vi "CalStruct_View V2.vi"(8 "error in":errorcluster) -> (0 "error out":errorcluster, 2 "calbuffer":u8[](array[numeric]), 3 "Return Code":i32)   [LabVIEW 2015]
doc: "Description:\nThis function will pass a copy of the calibration structure back to a host program. The host program must be able to parse the EEPROM structure (See Appendix 1).\nDetail:\nint CalStruct_View (\nchar * calbuffer );\n\nParameters:\nchar * calbuffer - Pointer to a character buffer of bytes (needs to be able to fit the EEPROM struct data, which is currently 332 bytes), which is loaded with the local EEPROM data from the DLL.\n\nReturn Values:\nThis function returns a 0 if the function completed successfully. A non-zero return code will indicate error."
uses:
  ScannerDiagDLL.dll
panel:
  out "CalData 2":T1
  out "CalData":T1
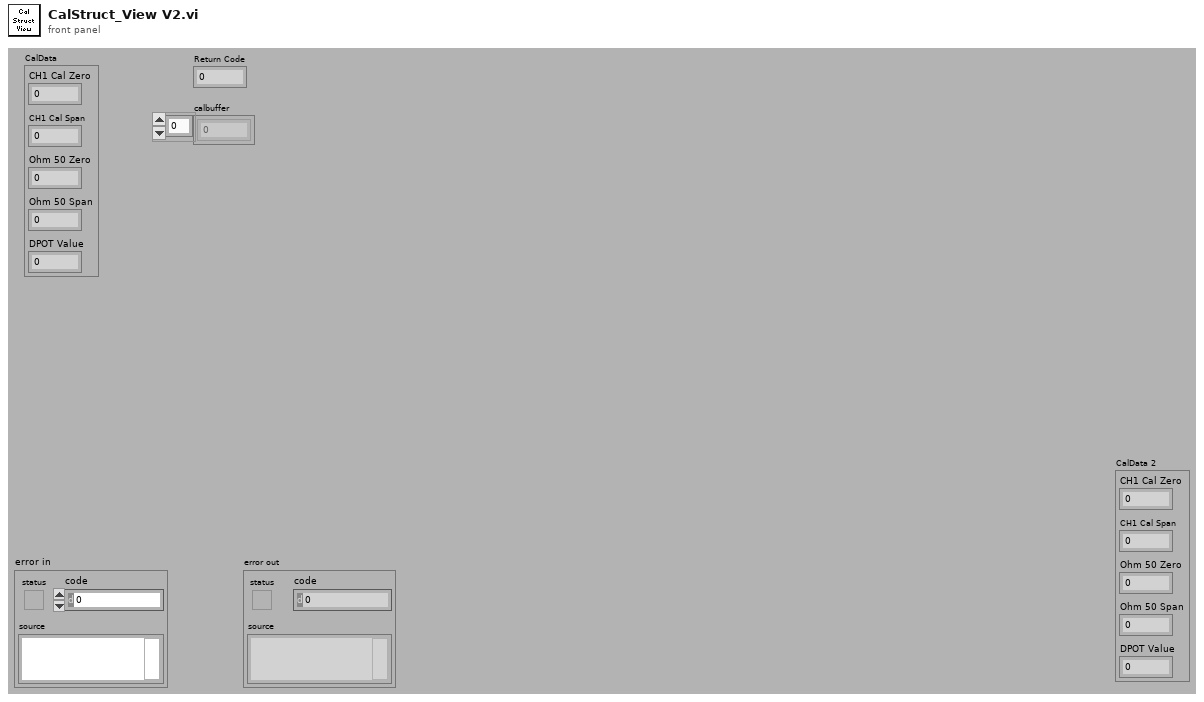
[diagram p1: front panel]
types:
  T1 = cluster{"CH1 Cal Zero ":u32, "CH1 Cal Span":u32, "Ohm 50 Zero ":u32, "Ohm 50 Span ":u32, "DPOT Value ":u32}
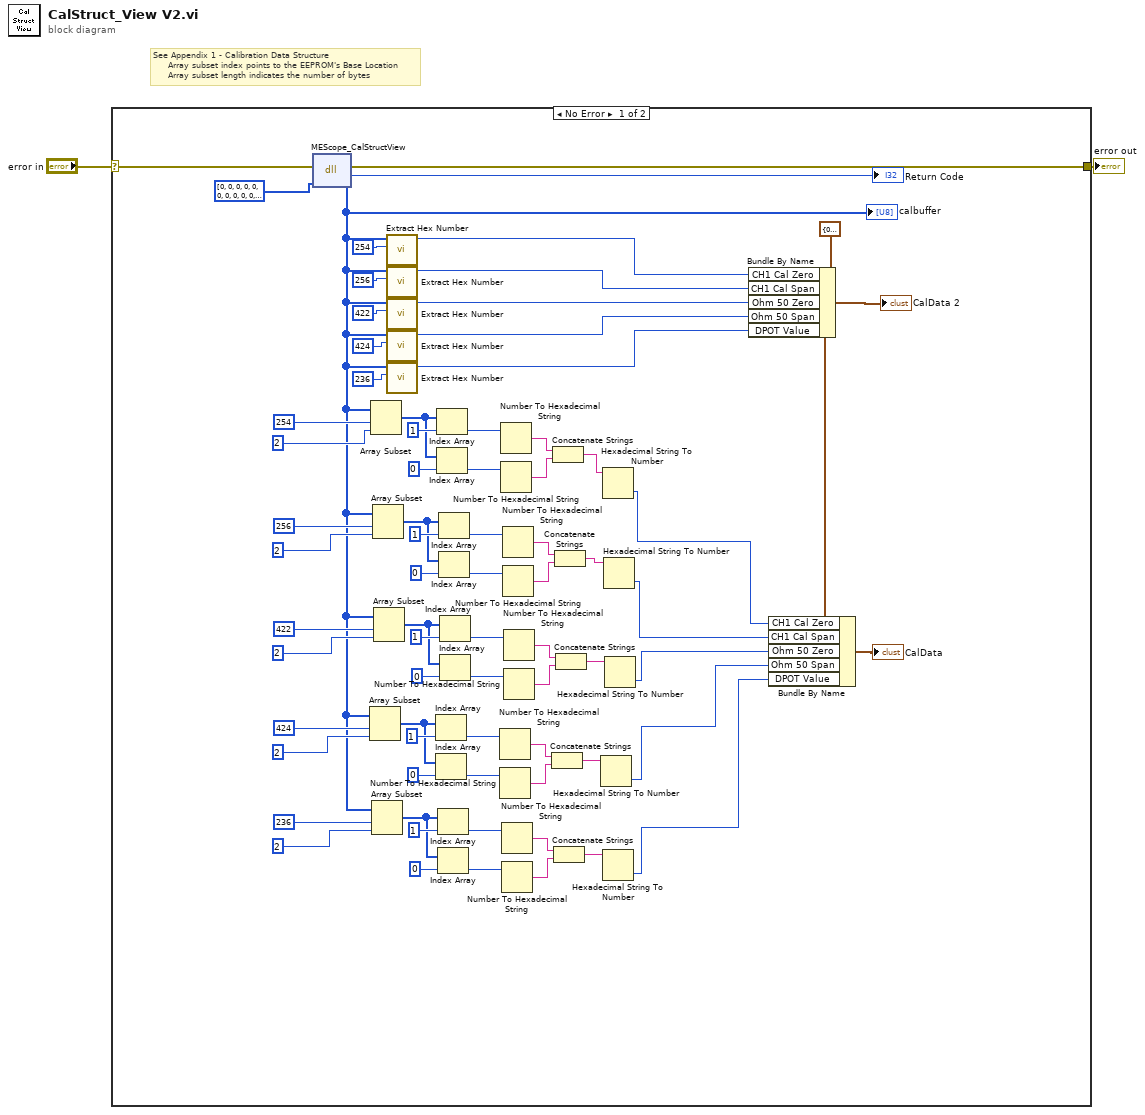
[diagram p0: block diagram]
diagram:
  # "See Appendix 1 - Calibration Data Structure\n     Array subset index points to the EEPROM's Base Location\n     Array subset length indicates the number of bytes"
  n1 = case shown="No Error" "error in" {
    selector: "error in" -> [w75 w76]
    tunnel: [w74 w76] -> w1
    frame No Error {
      w3 = T1 {"CH1 Cal Zero "=0, "CH1 Cal Span"=0, "Ohm 50 Zero "=0, "Ohm 50 Span "=0, "DPOT Value "=0} ("CalstructView")
      n2 = dll-call lib="C:/SNAPON/ModisEdge/TabletScope/Test Sequence/Code Modules/DLL/ScannerDiagDLL.dll" fn="MEScope_CalStructView"(error in=w75, "calbuffer"=u8[] [0, 0, 0, 0, 0, 0, 0, 0, 0, 0, 0, 0, 0, 0, 0, 0, 0, 0, 0, 0, 0, 0, 0, 0, 0, 0, 0, 0, 0, 0, 0, 0, 0, 0, 0, 0, 0, 0, 0, 0, 0, 0, 0, 0, 0, 0, 0, 0, 0, 0, 0, 0, 0, 0, 0, 0, 0, 0, 0, 0, 0, 0, 0, 0, 0, 0, 0, 0, 0, 0, 0, 0, 0, 0, 0, 0, 0, 0, 0, 0, 0, 0, 0, 0, 0, 0, 0, 0, 0, 0, 0, 0, 0, 0, 0, 0, 0, 0, 0, 0, 0, 0, 0, 0, 0, 0, 0, 0, 0, 0, 0, 0, 0, 0, 0, 0, 0, 0, 0, 0, 0, 0, 0, 0, 0, 0, 0, 0, 0, 0, 0, 0, 0, 0, 0, 0, 0, 0, 0, 0, 0, 0, 0, 0, 0, 0, 0, 0, 0, 0, 0, 0, 0, 0, 0, 0, 0, 0, 0, 0, 0, 0, 0, 0, 0, 0, 0, 0, 0, 0, 0, 0, 0, 0, 0, 0, 0, 0, 0, 0, 0, 0, 0, 0, 0, 0, 0, 0, 0, 0, 0, 0, 0, 0, 0, 0, 0, 0, 0, 0, 0, 0, 0, 0, 0, 0, 0, 0, 0, 0, 0, 0, 0, 0, 0, 0, 0, 0, 0, 0, 0, 0, 0, 0, 0, 0, 0, 0, 0, 0, 0, 0, 0, 0, 0, 0, 0, 0, 0, 0, 0, 0, 0, 0, 0, 0, 0, 0, 0, 0, 0, 0, 0, 0, 0, 0, 0, 0, 0, 0, 0, 0, 0, 0, 0, 0, 0, 0, 0, 0, 0, 0, 0, 0, 0, 0, 0, 0, 0, 0, 0, 0, 0, 0, 0, 0, 0, 0, 0, 0, 0, 0, 0, 0, 0, 0, 0, 0, 0, 0, 0, 0, 0, 0, 0, 0, 0, 0, 0, 0, 0, 0, 0, 0, 0, 0, 0, 0, 0, 0, 0, 0, 0, 0, 0, 0, 0, 0, 0, 0, 0, 0, 0, 0, 0, 0, 0, 0, 0, 0, 0, 0, 0, 0, 0, 0, 0, 0, 0, 0, 0, 0, 0, 0, 0, 0, 0, 0, 0, 0, 0, 0, 0, 0, 0, 0, 0, 0, 0, 0, 0, 0, 0, 0, 0, 0, 0, 0, 0, 0, 0, 0, 0, 0, 0, 0, 0, 0, 0, 0, 0, 0, 0, 0, 0, 0, 0, 0, 0, 0, 0, 0, 0, 0, 0, 0, 0, 0, 0, 0, 0, 0, 0, 0, 0, 0, 0, 0, 0, 0, 0, 0, 0, 0, 0, 0, 0, 0, 0, 0, 0, 0, 0, 0, 0, 0, 0, 0, 0, 0, 0, 0, 0, 0, 0, 0, 0, 0, 0, 0, 0, 0, 0, 0, 0, 0, 0, 0, 0, 0, 0, 0, 0, 0, 0, 0, 0, 0, 0, 0, 0, 0, 0, 0, 0, 0, 0, 0, 0, 0, 0, 0, 0, 0, 0, 0, 0, 0, 0, 0, 0, 0, 0, 0, 0, 0, 0, 0, 0, 0, 0, 0, 0, 0, 0, 0, 0, 0, 0, 0, 0, 0, 0, 0, 0, 0, 0, 0, 0, 0, 0, 0, 0, 0, 0, 0, 0, 0, 0, 0, 0, 0, 0, 0, 0, 0, 0, 0, 0, 0, 0, 0, 0, 0, 0, 0, 0, 0, 0, 0, 0, 0, 0, 0, 0, 0, 0, 0, 0, 0, 0, 0, 0, 0, 0, 0, 0, 0, 0, 0, 0, 0, 0, 0, 0, 0, 0, 0, 0, 0, 0, 0, 0, 0, 0, 0, 0, 0, 0, 0, 0, 0, 0, 0, 0, 0, 0, 0, 0, 0, 0]) -> (error out=w74:errorcluster, "return type"=→"Return Code":i32, "calbuffer"=w4:u8[])  [unwired: 2 in, 1 out]
      "calbuffer" <- w4
      n3 = Array Subset(array=w4, index=424, length=2) -> (w39:u8[])
      n4 = Array Subset(array=w4, index=254, length=2) -> (w67:u8[])
      n5 = Array Subset(array=w4, index=236, length=2) -> (w29:u8[])
      n6 = Array Subset(array=w4, index=256, length=2) -> (w59:u8[])
      n7 = Array Subset(array=w4, index=422, length=2) -> (w49:u8[])
      n8 = call "Extract Hex Number.vi"("index"=254, "unsigned byte array"=w4) -> ("Numeric"=w7:u16)  [unwired: 9 in]
      n9 = call "Extract Hex Number.vi"("index"=256, "unsigned byte array"=w4) -> ("Numeric"=w8:u16)  [unwired: 9 in]
      n10 = call "Extract Hex Number.vi"("index"=422, "unsigned byte array"=w4) -> ("Numeric"=w9:u16)  [unwired: 9 in]
      n11 = call "Extract Hex Number.vi"("index"=424, "unsigned byte array"=w4) -> ("Numeric"=w10:u16)  [unwired: 9 in]
      n12 = call "Extract Hex Number.vi"("index"=236, "unsigned byte array"=w4) -> ("Numeric"=w11:u16)  [unwired: 9 in]
      n13 = Index Array(array=w39, index=1) -> (element=w38:u8)
      n14 = Index Array(array=w39, index=0) -> (element=w37:u8)
      n15 = Index Array(array=w67, index=1) -> (element=w66:u8)
      n16 = Index Array(array=w67, index=0) -> (element=w65:u8)
      n17 = Index Array(array=w29, index=1) -> (element=w28:u8)
      n18 = Index Array(array=w29, index=0) -> (element=w27:u8)
      n19 = Index Array(array=w59, index=1) -> (element=w58:u8)
      n20 = Index Array(array=w59, index=0) -> (element=w57:u8)
      n21 = Index Array(array=w49, index=1) -> (element=w48:u8)
      n22 = Index Array(array=w49, index=0) -> (element=w47:u8)
      n23 = Number To Hexadecimal String(2:w38) -> (0:w36:string)  [unwired: 1 in]
      n24 = Number To Hexadecimal String(2:w37) -> (0:w35:string)  [unwired: 1 in]
      n25 = Number To Hexadecimal String(2:w66) -> (0:w63:string)  [unwired: 1 in]
      n26 = Number To Hexadecimal String(2:w65) -> (0:w62:string)  [unwired: 1 in]
      n27 = Number To Hexadecimal String(2:w28) -> (0:w26:string)  [unwired: 1 in]
      n28 = Number To Hexadecimal String(2:w27) -> (0:w25:string)  [unwired: 1 in]
      n29 = Number To Hexadecimal String(2:w58) -> (0:w56:string)  [unwired: 1 in]
      n30 = Number To Hexadecimal String(2:w57) -> (0:w55:string)  [unwired: 1 in]
      n31 = Number To Hexadecimal String(2:w48) -> (0:w46:string)  [unwired: 1 in]
      n32 = Number To Hexadecimal String(2:w47) -> (0:w45:string)  [unwired: 1 in]
      n33 = Concatenate Strings(w36, w35) -> (w33:string)
      n34 = Concatenate Strings(w63, w62) -> (w64:string)
      n35 = Concatenate Strings(w26, w25) -> (w23:string)
      n36 = Concatenate Strings(w56, w55) -> (w53:string)
      n37 = Concatenate Strings(w46, w45) -> (w43:string)
      n38 = Hexadecimal String To Number(string=w33) -> (number=w18:u32)  [unwired: 2 in, 1 out]
      n39 = Hexadecimal String To Number(string=w64) -> (number=w21:u32)  [unwired: 2 in, 1 out]
      n40 = Hexadecimal String To Number(string=w23) -> (number=w17:u32)  [unwired: 2 in, 1 out]
      n41 = Hexadecimal String To Number(string=w53) -> (number=w20:u32)  [unwired: 2 in, 1 out]
      n42 = Hexadecimal String To Number(string=w43) -> (number=w19:u32)  [unwired: 2 in, 1 out]
      n43 = Bundle By Name(cluster=w3, "CH1 Cal Zero"=w7, "CH1 Cal Span"=w8, "Ohm 50 Zero"=w9, "Ohm 50 Span"=w10, "DPOT Value"=w11) -> (→"CalData 2":T1)
      n44 = Bundle By Name(cluster=w3, "CH1 Cal Zero"=w21, "CH1 Cal Span"=w20, "Ohm 50 Zero"=w19, "Ohm 50 Span"=w18, "DPOT Value"=w17) -> (→"CalData":T1)
    }
    frame Error {
    }
  }
  "error out" <- w1
